vi "Calculate angle.vi"(10 "XY Coordinates":i32[](array[numeric])) -> (1 "Angle (deg)":dbl)   [LabVIEW 2017]
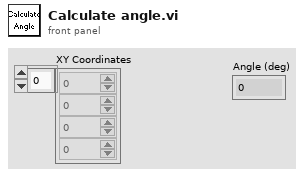
[diagram p1: front panel]
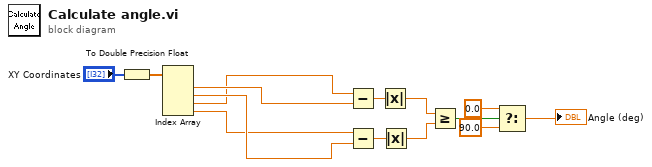
[diagram p0: block diagram]
diagram:
  n1 = To Double Precision Float(number="XY Coordinates") -> (double precision float=w2:dbl[])
  n2 = Index Array(array=w2) -> (element #1=w7:dbl, element #2=w6:dbl, element #3=w5:dbl, element #4=w4:dbl)  [unwired: 4 in]
  n3 = Subtract(x=w5, y=w7) -> (x-y=w10:dbl)
  n4 = Subtract(x=w4, y=w6) -> (x-y=w11:dbl)
  n5 = Absolute Value(x=w10) -> (abs(x)=w9:dbl)
  n6 = Absolute Value(x=w11) -> (abs(x)=w8:dbl)
  n7 = Greater Or Equal?(x=w9, y=w8) -> (x >= y?=w1:bool)
  n8 = Select(t=0.0, s=w1, f=90.0) -> (s? t:f=→"Angle (deg)":dbl)
